vi "Write Single Coil.vi"(8 "error in (no error)":errorcluster, 9 "coil value":bool, 10 "address":u16, 11 "Modbus master in":refnum<class "Modbus Master.lvclass">) -> (0 "error out":errorcluster, 3 "Modbus master out":refnum<class "Modbus Master.lvclass">)   [LabVIEW 2018, in "Modbus Master.lvclass"]
doc: "Writes a value to a single coil."
uses:
  Modbus Master.lvclass
  C:/Program Files (x86)/National Instruments/LabVIEW 2018/vi.lib/Modbus/subvis/Modbus API/Modbus API.lvclass
  Modbus API.lvclass/Modbus API.ctl
  Modbus Master.lvclass/Modbus Master.ctl
  Network Master.lvclass
  C:/Program Files (x86)/National Instruments/LabVIEW 2018/vi.lib/Modbus/subvis/Protocol/Interfaces/Network Protocol/Network Protocol.lvclass
  Transmission Data Unit.lvclass
  Master Function Definition.lvlib
  Modbus API.lvclass
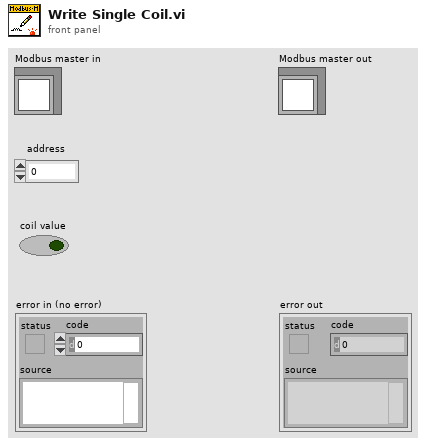
[diagram p1: front panel]
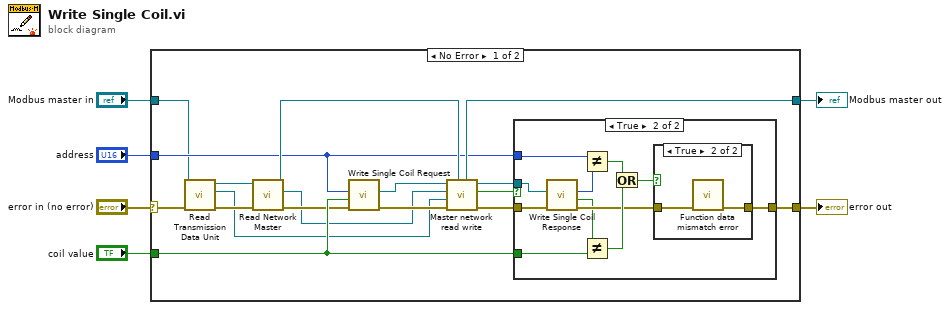
[diagram p0: block diagram]
diagram:
  n1 = case shown="No Error" "error in (no error)" {
    selector: "error in (no error)" -> [w7 w40]
    tunnel: "Modbus master in" -> [w8 w39]
    tunnel: [w22 w40] -> w3
    tunnel: [w17 w39] -> w2
    tunnel: "address" -> [w10 _]
    tunnel: "coil value" -> [w21 _]
    frame No Error {
      n2 = call "Read Transmission Data Unit.vi"("error in (no error)"=w7, "Modbus instance in"=w8) -> ("error out"=w15:errorcluster, "transmission data unit"=w11:refnum<class "Transmission Data Unit.lvclass">, "Modbus instance out"=w16:refnum<class "Modbus Master.lvclass">)  [unwired: 7 in]
      n3 = call "Read Network Master.vi"("error in (no error)"=w15, "Modbus master in"=w16) -> ("error out"=w14:errorcluster, "network master"=w12:refnum<class "Network Master.lvclass">, "Modbus master out"=w13:refnum<class "Modbus Master.lvclass">)  [unwired: 7 in]
      n4 = call "Write Single Coil Request.vi"("error in (no error)"=w14, "coil value"=w21, "starting address"=w10) -> ("error out"=w23:errorcluster, "Modbus data unit out"=w19:refnum<class "Modbus Data Unit (PDU).lvclass">)  [unwired: 7 in]
      n5 = call "Master network read write.vi"("Modbus master in"=w13, "error in (no error)"=w23, "transmission data unit in"=w11, "network master in"=w12, "Modbus data unit in"=w19) -> ("error out"=w20:errorcluster, "PDU valid?"=w9:bool, "Modbus data unit out"=w18:refnum<class "Modbus Data Unit (PDU).lvclass">, "Modbus master out"=w17:refnum<class "Modbus Master.lvclass">)  [unwired: 3 in]
      n6 = case shown="True" w9 {
        tunnel: [w24 w34] -> w22
        tunnel: w21 -> [_ w26]
        tunnel: w20 -> [w24 w30]
        tunnel: w18 -> [_ w29]
        tunnel: w10 -> [_ w27]
        frame False {
        }
        frame True {
          n7 = call "Write Single Coil Response.vi"("error in (no error)"=w30, "Modbus data unit in"=w29) -> ("error out"=w28:errorcluster, "coil value"=w25:bool, "address"=w31:u16)  [unwired: 7 in]
          n8 = Not Equal?(x=w27, y=w31) -> (x != y?=w33:bool)
          n9 = Not Equal?(x=w25, y=w26) -> (x != y?=w32:bool)
          n10 = Or(x=w33, y=w32) -> (x .or. y?=w35:bool)
          n11 = case shown="True" w35 {
            tunnel: [w36 w38] -> w34
            tunnel: w28 -> [w36 w37]
            frame False {
            }
            frame True {
              n12 = call "Function data mismatch error.vi"("error in (no error)"=w37) -> ("error out"=w38:errorcluster)  [unwired: 10 in]
            }
          }
        }
      }
    }
    frame Error {
    }
  }
  "error out" <- w3
  "Modbus master out" <- w2
